vi "tree_ctl_selection.vi"() -> ()   [LabVIEW 2016]
uses:
  <userlib>/LevyLab/XY Utilities/xy_utilities.lvlib
panel:
  out "Array 2":string[][](array[string])
  out "Array":string[][](array[string])
  out "should be all ops to complete":string[](array[string])
  in  "input data":dbl[][](graph)
  out "processed data":dbl[][](graph)
  out "values":string[](array[string])
  out "properties":string[](array[string])
  out "indentations":i32[](array[numeric])
  in  "Operations Palette":string(tree)
  in  "Operations to Perform":string(tree)
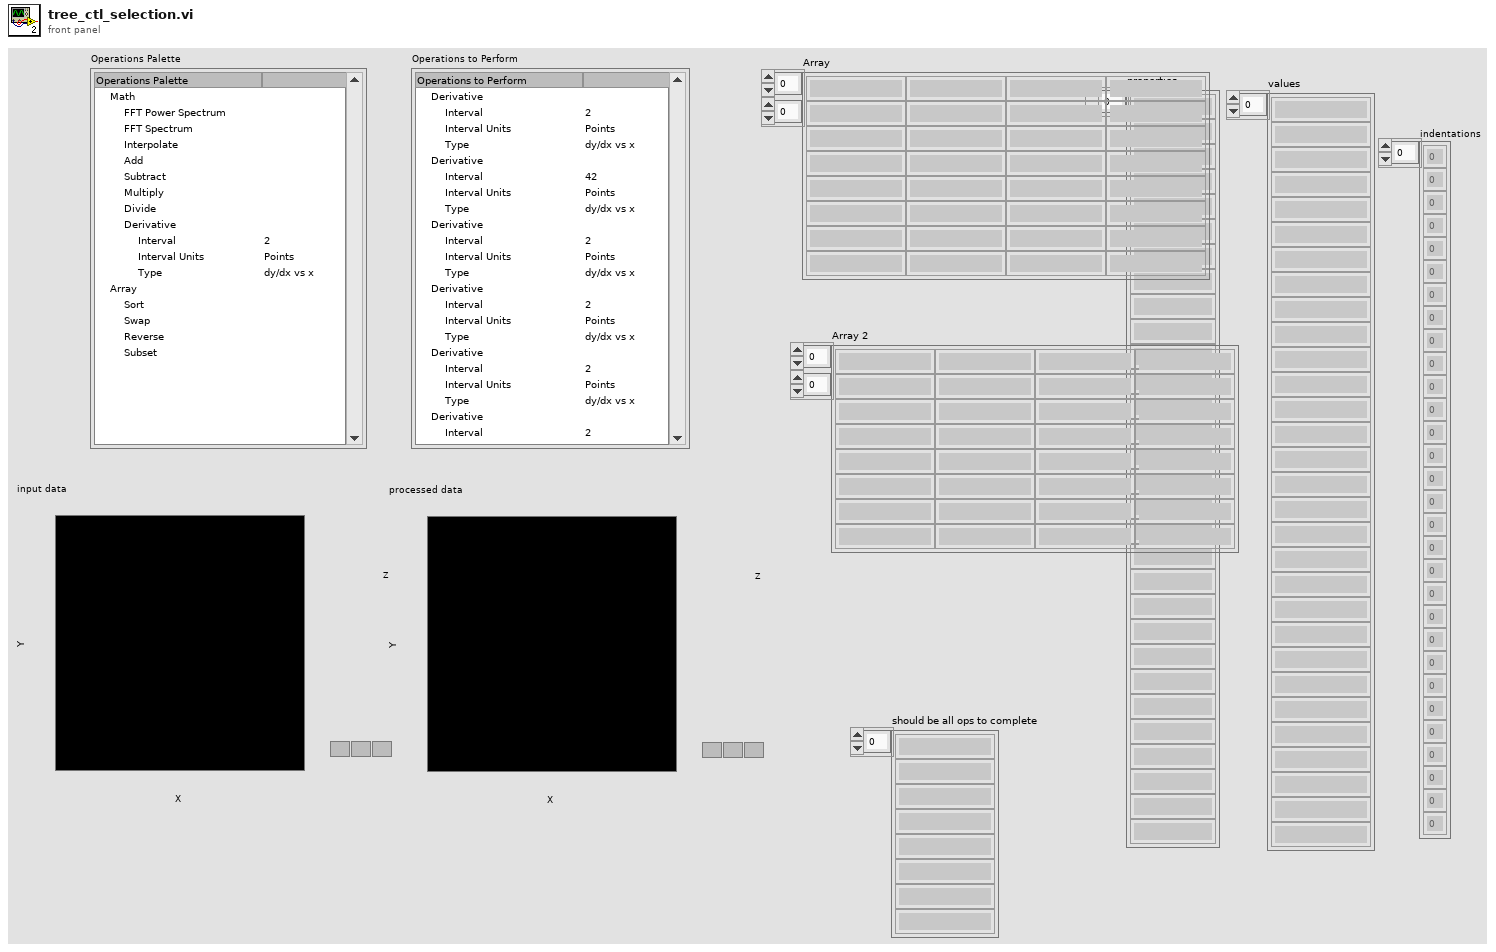
[diagram p1: front panel]
types:
  T1 = cluster{"Interval Units":enum16{"Points", "Data"}, "Interval":dbl, "Type":enum16{"dy/dx vs x", "dx/dy vs y"}}
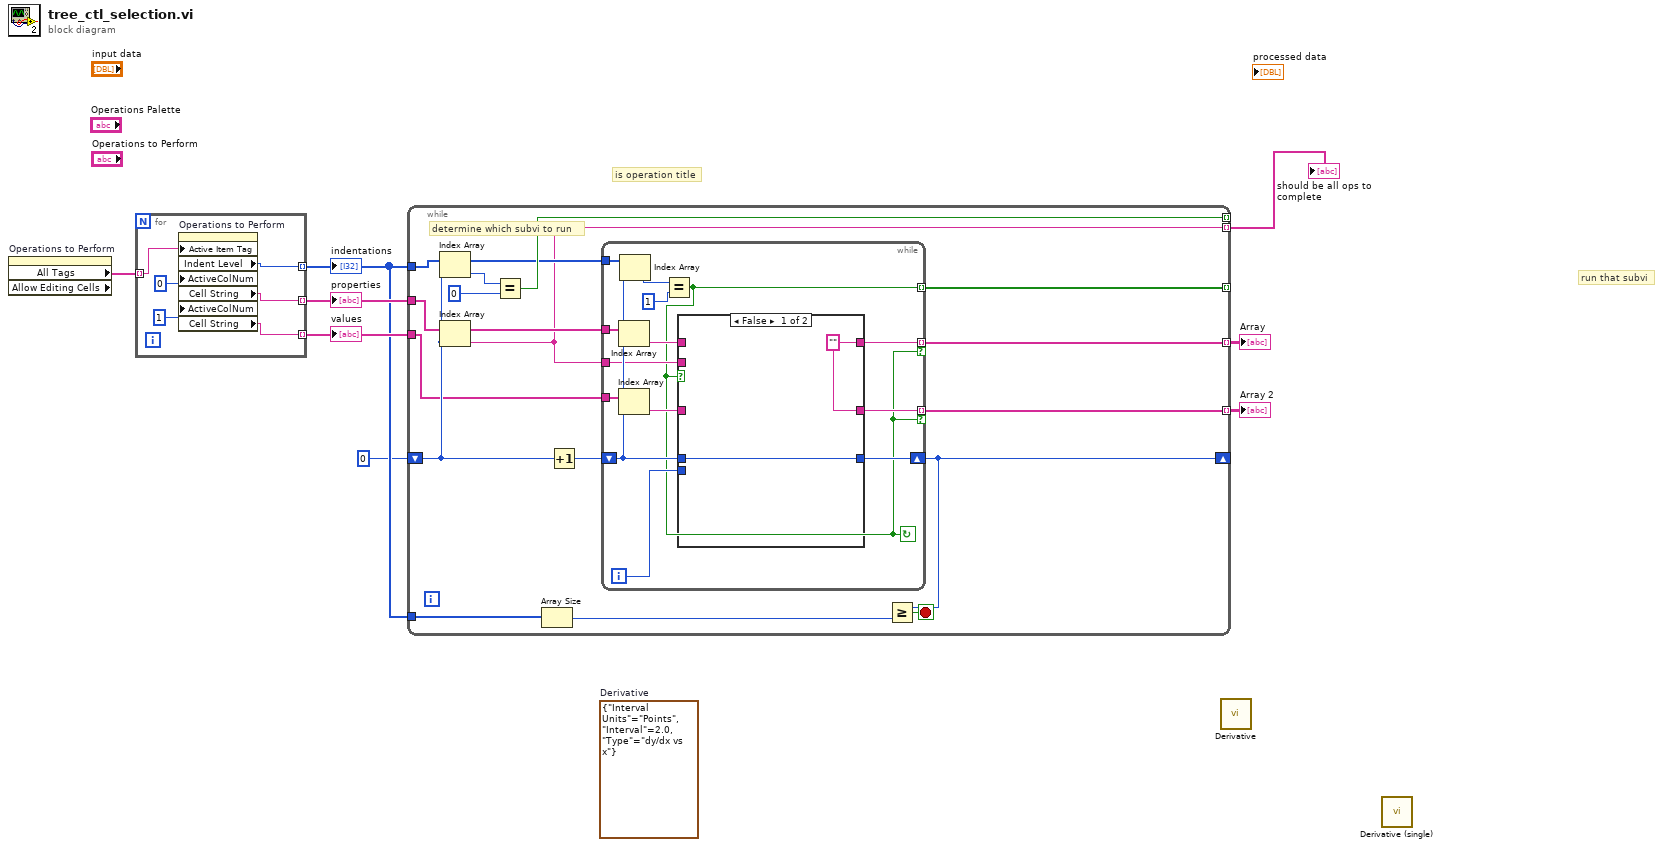
[diagram p0: block diagram]
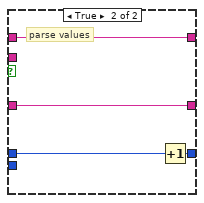
[diagram p2: hidden frame]
diagram:
  (unwired) T1 {"Interval Units"=enum."Points", "Interval"=2.0, "Type"=enum."dy/dx vs x"}  # Derivative
  # "is operation title"
  # "run that subvi"
  n1 = property on="Operations to Perform" class="Tree (strict)" props=["All Tags", "Allow Editing Cells"]() -> ("All Tags"=w6:string[])  [unwired: 2 in, 3 out]
  n2 = for {
    tunnel: w6 -> [w13] mode=indexing
    tunnel: [w14] -> w5 mode=indexing
    tunnel: [w10] -> w8 mode=indexing
    tunnel: [w9] -> w7 mode=indexing
    n3 = property on="Operations to Perform" class="Tree (strict)"("Active Item Tag"=w13, "ActiveColNum"=0 ("Active Cell:Active Column Number"), "ActiveColNum"=1 ("Active Cell:Active Column Number")) -> ("Indent Level"=w14:i32, "Cell String"=w10:string, "Cell String"=w9:string)  [unwired: 2 in, 2 out]
  }
  "indentations" <- w5
  "properties" <- w8
  "values" <- w7
  n4 = while {
    tunnel: w5 -> [w22]
    tunnel: w8 -> [w20]
    tunnel: w7 -> [w18]
    tunnel: w5 -> [w30]
    shift-right: [w19] -> _
    shift-left: 0 -> [w24]
    tunnel: [w25] -> _ mode=indexing
    tunnel: [w17] -> w3 mode=indexing
    tunnel: [w21] -> _ mode=indexing
    tunnel: [w16] -> w2 mode=indexing
    tunnel: [w15] -> w1 mode=indexing
    stop <- w28 stop-if-true
    # "determine which subvi to run"
    n5 = Index Array(array=w22, index=w24) -> (element=w26:i32)
    n6 = Index Array(array=w20, index=w24) -> (element=w17:string)
    n7 = Equal?(x=w26, y=0) -> (x = y?=w25:bool)
    n8 = Array Size(array=w30) -> (size(s)=w29:i32)
    n9 = Increment(x=w24) -> (x+1=w23:i32)
    n10 = while {
      shift-right: [w44] -> w19
      shift-left: w23 -> [w39]
      tunnel: w22 -> [w43]
      tunnel: [w31] -> w21 mode=indexing
      tunnel: w20 -> [w40]
      tunnel: w18 -> [w38]
      tunnel: w17 -> [w34]
      tunnel: [w33] -> w16 mode=indexing if=w31
      tunnel: [w32] -> w15 mode=indexing if=w31
      i -> [w35]
      stop <- w31 continue-if-true
      n11 = Index Array(array=w40, index=w39) -> (element=w36:string)
      n12 = Index Array(array=w38, index=w39) -> (element=w37:string)
      n13 = Index Array(array=w43, index=w39) -> (element=w41:i32)
      n14 = Equal?(x=w41, y=1) -> (x = y?=w31:bool)
      n15 = case shown="False" w31 {
        tunnel: [w46 w50] -> w44
        tunnel: w39 -> [w46 w49]
        tunnel: w37 -> [_ w47]
        tunnel: w36 -> [_ w48]
        tunnel: w35 -> [_ _]
        tunnel: w34 -> [_ _]
        tunnel: [w45 w48] -> w33
        tunnel: [w45 w47] -> w32
        frame False {
          w45 = ""
        }
        frame True {
          # "parse values"
          n16 = Increment(x=w49) -> (x+1=w50:i32)
        }
      }
    }
    n17 = Greater Or Equal?(x=w19, y=w29) -> (x >= y?=w28:bool)
  }
  "should be all ops to complete" <- w3
  "Array" <- w2
  "Array 2" <- w1
  n18 = call-poly <userlib>:"Derivative.vi"() -> ()  [unwired: 9 in, 3 out]
  n19 = call <userlib>:"Derivative (single).vi"() -> ()  [unwired: 9 in, 3 out]
